vi "test_Basic Deployment.vi"(8 "error in (no error)":errorcluster, 11 "TestCase in":refnum<class "Common System Tests.lvclass">) -> (0 "error out":errorcluster, 3 "TestCase out":refnum<class "Common System Tests.lvclass">)   [LabVIEW 2019, in "Common System Tests.lvclass"]
uses:
  Common System Tests.lvclass
  C:/Dev/ni-master/niveristand-custom-device-testing-tools/VeriStandTestCase/VeriStandTestCase.lvclass
  ni-master/niveristand-custom-device-testing-tools/VeriStandTestUtilities/SystemDefinitionInformation.ctl
  ni-master/niveristand-custom-device-testing-tools/VeriStandTestUtilities/TargetInformation.ctl
  ni-master/niveristand-custom-device-testing-tools/VeriStandTestUtilities/ChassisInformation.ctl
  <vilib>/addons/_JKI Toolkits/VI Tester/TestCase.llb/TestCase.lvclass
  C:/Program Files (x86)/National Instruments/LabVIEW 2019/vi.lib/addons/_JKI Toolkits/VI Tester/TestCase.llb/TestCase.lvclass
  ni-master/niveristand-custom-device-testing-tools/VeriStandTestUtilities/VeriStandTestUtilities.lvlib
panel:
  out "System Definition Information":T1
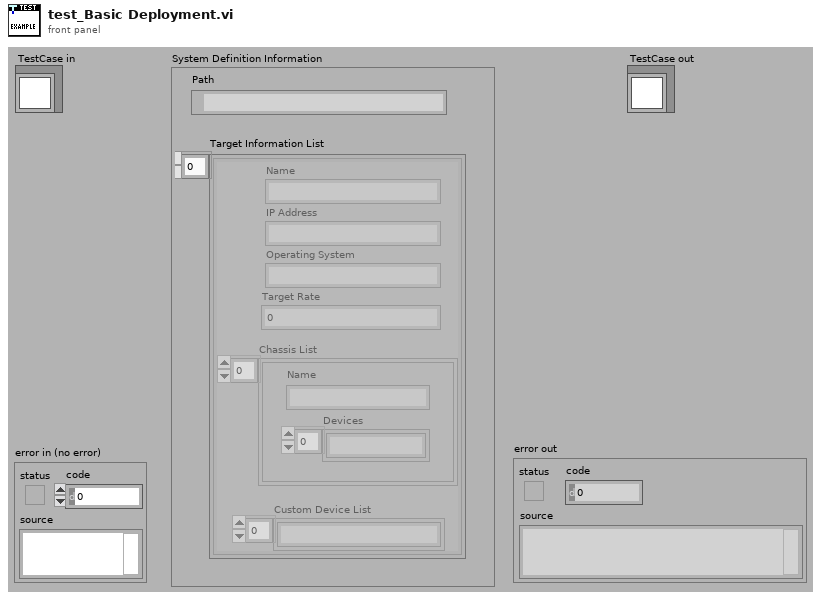
[diagram p1: front panel]
types:
  T1 = typedef "VeriStandTestUtilities.lvlib/SystemDefinitionInformation.ctl" = cluster{"Path":path, "Target Information List":T2[]}
  T2 = typedef "VeriStandTestUtilities.lvlib/TargetInformation.ctl" = cluster{"Name":string, "IP Address":string, "Operating System":string, "Target Rate":dbl, "Chassis List":T3[], "Custom Device List":string[]}
  T3 = typedef "VeriStandTestUtilities.lvlib/ChassisInformation.ctl" = cluster{"Name":string, "Devices":string[]}
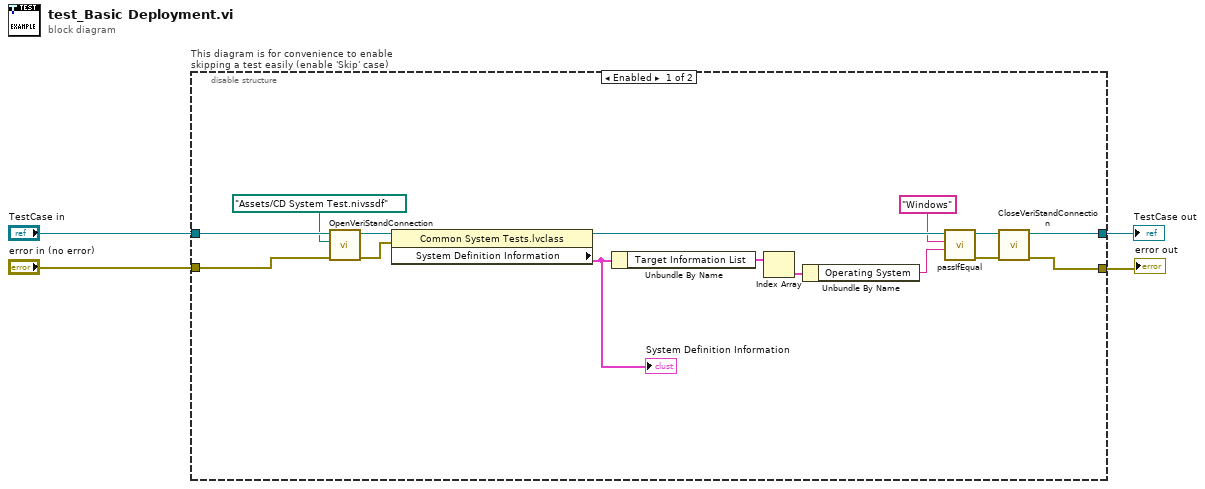
[diagram p0: block diagram]
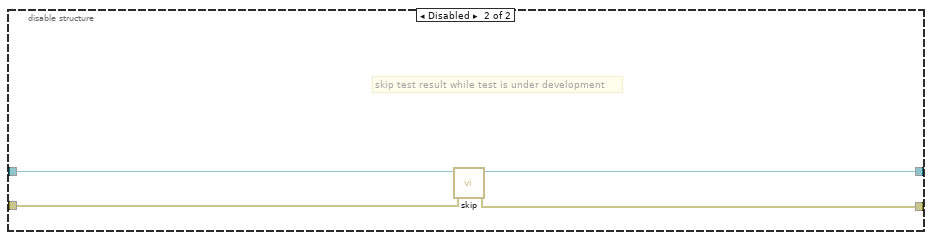
[diagram p2: hidden frame]
diagram:
  n1 = disable-structure "This diagram is for convenience to enable skipping a test easily (enable 'Skip' case)" shown="Enabled" {
    disable-tunnel: "TestCase in" -> [w15 w23]
    disable-tunnel: [w16 w21] -> w1
    disable-tunnel: [w17 w22] -> w3
    disable-tunnel: "error in (no error)" -> [w13 w20]
    frame Enabled {
      n2 = call-dynamic "OpenVeriStandConnection.vi"("error in (no error)"=w13, "System Definition File"=path "Assets/CD System Test.nivssdf", "VeriStand Test Case in"=w15) -> ("error out"=w12:errorcluster, "VeriStand Test Case out"=w14:refnum<class "Common System Tests.lvclass">)  [unwired: 6 in, 1 out]
      n3 = property class="Common System Tests.lvclass"(reference=w14, error in=w12) -> (reference out=w11:refnum<class "Common System Tests.lvclass">, "System Definition Information"=w7:T1)  [unwired: 1 out]
      "System Definition Information" <- w7
      n4 = Unbundle By Name(w7) -> ("Target Information List"=w9:T2[])
      n5 = Index Array(array=w9) -> (element=w8:T2)  [unwired: 1 in]
      n6 = Unbundle By Name(w8) -> ("Operating System"=w6:string)
      n7 = call-dynamic "passIfEqual.vi"("y"=w6, "x"="Windows" ("Operating System"), "TestCase in"=w11) -> ("error out"=w18:errorcluster, "TestCase out"=w19:refnum<class "Common System Tests.lvclass">)  [unwired: 7 in]
      n8 = call-dynamic "CloseVeriStandConnection.vi"("error in (no error)"=w18, "VeriStand Test Case in"=w19) -> ("error out"=w17:errorcluster, "VeriStand Test Case out"=w16:refnum<class "Common System Tests.lvclass">)  [unwired: 8 in]
    }
    frame Disabled {
      # "skip test result while test is under development"
      n9 = call <vilib>:"skip.vi"("error in (no error)"=w20, "TestCase in"=w23) -> ("error out"=w22:errorcluster, "TestCase out"=w21:refnum<class "Common System Tests.lvclass">)  [unwired: 8 in]
    }
  }
  "error out" <- w3
  "TestCase out" <- w1
